vi "ps10.vi"(0 "Image In":T1, 1 "Template File Path (Geometric Matching 1)":path=path "C:/Users/M.H.Najafi/Desktop/pictures/PPT/pattern/ps10.png", 7 "error in":errorcluster) -> (20 "Image Out":T1, 21 "Matches (Geometric Matching 1)":T2[](array[typedef]) {"Correlation Score" format="%.2f"; "Target Template Curve Score" format="%.2f"; "Template Target Curve Score" format="%.2f"; "Bounding Box"."y" format="%.2f"; "Bounding Box"."x" format="%.2f"; "Position"."y" format="%.2f"; "Position"."x" format="%.2f"; "Score" format="%.2f"; "Scale" format="%.2f"; "Angle" format="%.2f"; "Occlusion %" format="%.2f"}, 27 "error out":errorcluster)   [LabVIEW 2017]
uses:
  <vilib>/vision/Image Controls.llb/IMAQ Image.ctl
  <vilib>/vision/Pattern Matching.llb/IMAQ GM Match Report.ctl
  <vilib>/vision/Pattern Matching.llb/IMAQ Curve Parameters.ctl
  <vilib>/vision/Pattern Matching.llb/IMAQ Match Range Setting.ctl
  <vilib>/vision/NI_Vision_Development_Module.lvlib
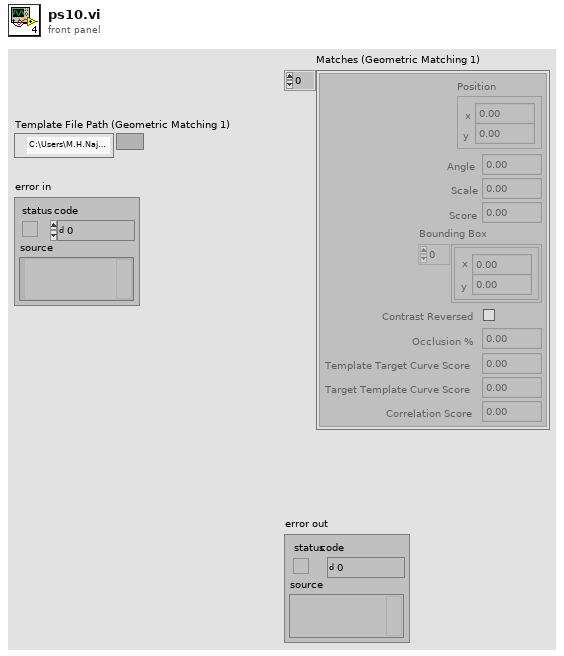
[diagram p1: front panel]
types:
  T1 = typedef "IMAQ Image.ctl" = refnum<image>
  T2 = typedef "IMAQ GM Match Report.ctl" = cluster{"Position":cluster{"x":sgl, "y":sgl}, "Angle":sgl, "Scale":sgl, "Score":sgl, "Bounding Box":cluster{"x":sgl, "y":sgl}[], "Contrast Reversed":bool, "Occlusion %":sgl, "Template Target Curve Score":sgl, "Target Template Curve Score":sgl, "Correlation Score":sgl}
  T3 = typedef "IMAQ Curve Parameters.ctl" = cluster{"Extraction Mode":u32, "Edge Threshold":i32, "Edge Filter Size":u32, "Min Length":i32, "Row Search Step Size":i32, "Col Search Step Size":i32, "Max Endpoint Gap":i32, "Closed":bool, "Subpixel":bool}
  T4 = typedef "IMAQ Match Range Setting.ctl" = cluster{"Match Constraints":u32, "Min":dbl, "Max":dbl}
  T5 = cluster{"Curve Parameters":T3, "Match Mode":cluster{"Rotation":bool, "Scale":bool, "Occlusion":bool, "Reserved 1":bool, "Reserved 2":bool, "Reserved 3":bool}, "Range Settings":T4[], "Number of Matches":i32, "Minimum Match Score":sgl, "SubPixel Accuracy":bool, "Adv. Geometric Match Options 2":cluster{"Setup Data Item":u16, "Item Value":dbl}[]}
  T6 = cluster{"Global Rectangle":i32[], "Contours":cluster{"ID":enum32{"External", "Internal"}, "Type":u32, "Coordinates":i32[]}[]}
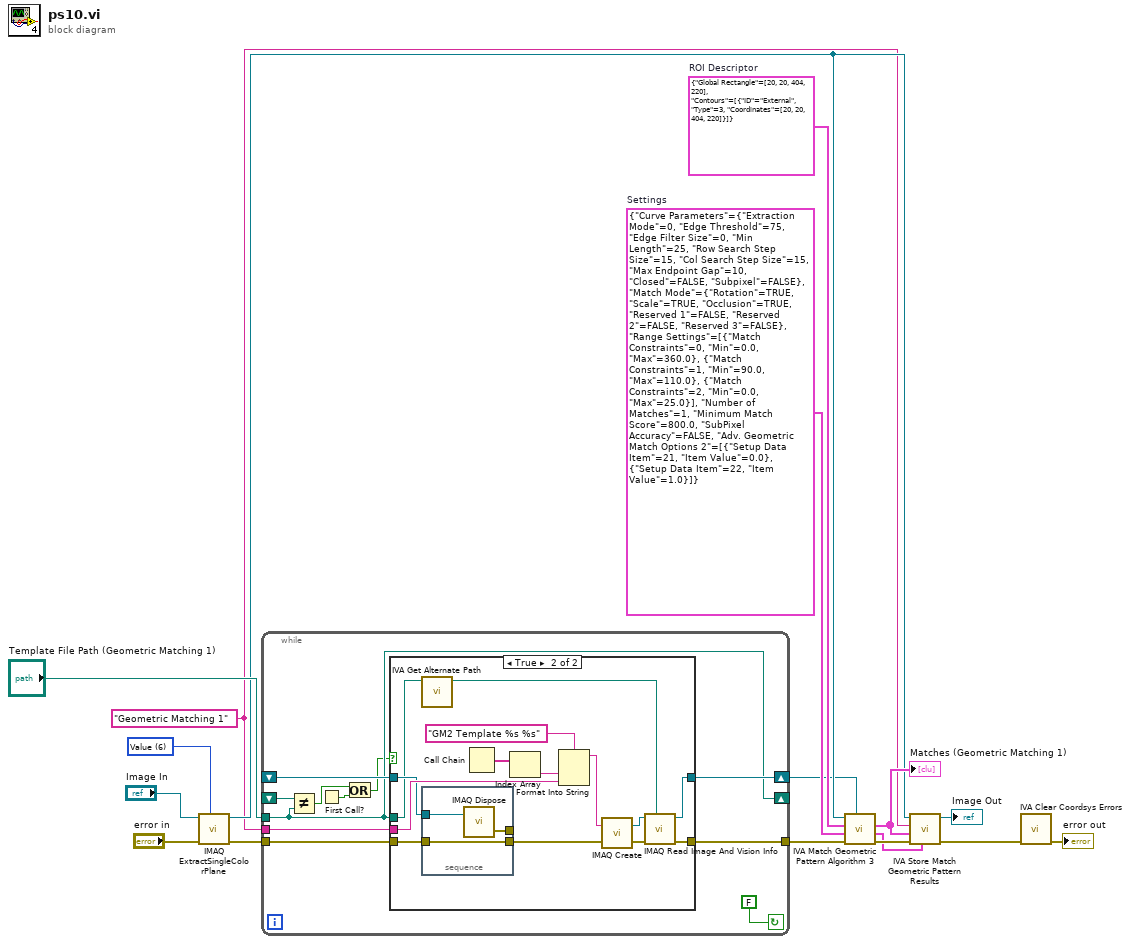
[diagram p0: block diagram]
diagram:
  w6 = T5 {"Curve Parameters"={"Extraction Mode"=0, "Edge Threshold"=75, "Edge Filter Size"=0, "Min Length"=25, "Row Search Step Size"=15, "Col Search Step Size"=15, "Max Endpoint Gap"=10, "Closed"=FALSE, "Subpixel"=FALSE}, "Match Mode"={"Rotation"=TRUE, "Scale"=TRUE, "Occlusion"=TRUE, "Reserved 1"=FALSE, "Reserved 2"=FALSE, "Reserved 3"=FALSE}, "Range Settings"=[{"Match Constraints"=0, "Min"=0.0, "Max"=360.0}, {"Match Constraints"=1, "Min"=90.0, "Max"=110.0}, {"Match Constraints"=2, "Min"=0.0, "Max"=25.0}], "Number of Matches"=1, "Minimum Match Score"=800.0, "SubPixel Accuracy"=FALSE, "Adv. Geometric Match Options 2"=[{"Setup Data Item"=21, "Item Value"=0.0}, {"Setup Data Item"=22, "Item Value"=1.0}]}  # Settings
  w5 = "Geometric Matching 1" ("Step Name")
  w13 = T6 {"Global Rectangle"=[20, 20, 404, 220], "Contours"=[{"ID"=enum."External", "Type"=3, "Coordinates"=[20, 20, 404, 220]}]}  # ROI Descriptor
  w17 = 6 items=["Red", "Green", "Blue", "Hue", "Saturation", "Luminance", "Value", "Intensity"] ("Color Plane")
  n1 = call "IMAQ ExtractSingleColorPlane"("Color Plane"=w17, "error in (no error)"="error in", "Image Src"="Image In") -> ("error out"=w8:errorcluster, "Image Dst Out"=w7:T1)  [unwired: 1 in, 6 out]
  n2 = while {
    shift-right: [w28] -> w3
    shift-left: _ -> [w27]
    tunnel: [w25] -> w4
    tunnel: w8 -> [w24]
    tunnel: "Template File Path (Geometric Matching 1)" -> [w21]
    tunnel: w5 -> [w23]
    shift-right: [w21] -> _
    shift-left: _ -> [w22]
    stop <- FALSE continue-if-true
    n3 = Not Equal?(x=w22, y=w21) -> (x != y?=w19:bool)
    n4 = First Call?() -> (First Call?: T/F=w20:bool)
    n5 = Or(x=w19, y=w20) -> (x .or. y?=w18:bool)
    n6 = case shown="True" w18 {
      tunnel: [w30 w42] -> w28
      tunnel: w27 -> [w30 w34]
      tunnel: [w29 w39] -> w25
      tunnel: w24 -> [w29 w35]
      tunnel: w23 -> [_ w36]
      tunnel: w21 -> [_ w33]
      frame False {
      }
      frame True {
        n7 = call <vilib>:"IVA Get Alternate Path.vi"("Path In"=w33) -> ("Path Out"=w32:path)  [unwired: 10 out]
        n8 = stacked-sequence {
          tunnel: w35 -> [w47]
          tunnel: w34 -> [w46]
          tunnel: [w47] -> w31
          tunnel: [w45] -> _
          frame #0 {
            n9 = call "IMAQ Dispose"("Image"=w46) -> ("error out"=w45:errorcluster)  [unwired: 2 in, 3 out]
          }
        }
        n10 = Call Chain() -> (call chain=w38:string[])
        n11 = Index Array(array=w38) -> (element=w37:string)  [unwired: 1 in]
        n12 = Format Into String(format string="GM2 Template %s %s" ("Image Name"), w37, w36) -> (resulting string=w44:string)  [unwired: 2 in, 1 out]
        n13 = call "IMAQ Create"("Image Name"=w44, "error in (no error)"=w31) -> ("New Image"=w41:T1, "error out"=w40:errorcluster)  [unwired: 2 in, 1 out]
        n14 = call "IMAQ Read Image And Vision Info"("File Path"=w32, "error in (no error)"=w40, "Image"=w41) -> ("error out"=w39:errorcluster, "Image Out"=w42:T1)  [unwired: 1 in, 6 out]
      }
    }
  }
  n15 = call <vilib>:"IVA Match Geometric Pattern Algorithm 3.vi"("Template"=w3, "error in (no error)"=w4, "Settings"=w6, "ROI Descriptor"=w13, "Image"=w7) -> ("error out"=w11:errorcluster, "Calibrated Matches"=w9:T2[], "Matches"=w10:T2[])  [unwired: 4 out]
  "Matches (Geometric Matching 1)" <- w10
  n16 = call <vilib>:"IVA Store Match Geometric Pattern Results.vi"("Calibrated Matches"=w9, "error in (no error)"=w11, "Matches"=w10, "Step Name"=w5, "Image in"=w7) -> ("error out"=w2:errorcluster, "Image dup"=→"Image Out":T1)  [unwired: 5 out]
  n17 = call <vilib>:"IVA Clear Coordsys Errors.vi"("error in (no error)"=w2) -> ("error out"=→"error out":errorcluster)  [unwired: 10 in]
